vi "Timeout.vi"(8 "error in (no error)":errorcluster, 11 "State Machine Actor in":refnum<class "State Machine Actor.lvclass">) -> (0 "error out":errorcluster, 3 "State Machine Actor out":refnum<class "State Machine Actor.lvclass">)   [LabVIEW 2024, in "State Machine Actor.lvlib" / "State Machine Actor.lvclass"]
uses:
  State Machine Actor.lvclass
  State Machine Actor.lvclass/State Machine Actor.ctl
  <vilib>/ActorFramework/Actor/Actor.lvclass/Actor.ctl
  <vilib>/ActorFramework/Message Enqueuer/Message Enqueuer.lvclass/Message Enqueuer.ctl
  _State Machine Actor/_State Machine Actor/_State Machine Actor.lvclass
  Timed Out/Timed Out/Timed Out.lvclass
  <vilib>/ActorFramework/Actor/Actor.lvclass
  <vilib>/ActorFramework/Message Enqueuer/Message Priority.ctl
  <vilib>/ActorFramework/Message Enqueuer/Message Enqueuer.lvclass
  State Machine Actor Messages/Timeout Msg/Timeout Msg.lvclass
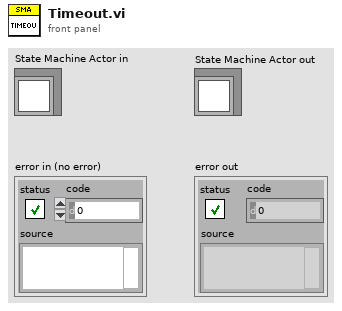
[diagram p1: front panel]
types:
  T1 = typedef "Actor Framework.lvlib/Message Enqueuer.lvclass/Message Priority.ctl" = enum16{"Low", "Normal", "High"}
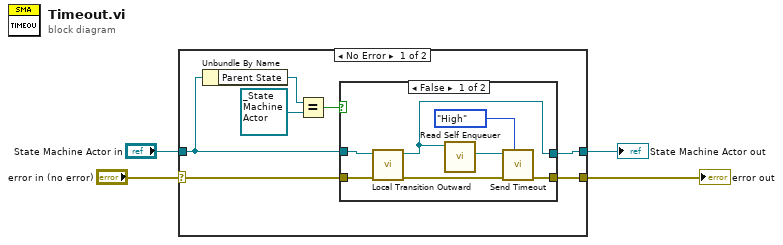
[diagram p0: block diagram]
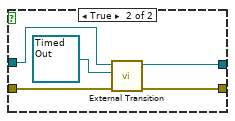
[diagram p2: hidden frame]
diagram:
  n1 = case shown="No Error" "error in (no error)" {
    selector: "error in (no error)" -> [w5 w25]
    tunnel: "State Machine Actor in" -> [w8 w24]
    tunnel: [w7 w24] -> w1
    tunnel: [w6 w25] -> w3
    frame No Error {
      n2 = Unbundle By Name(w8) -> ("Parent State"=w11:refnum<class "_State Machine Actor.lvclass">)
      n3 = Equal?(x=w11, y=refnum<class "_State Machine Actor.lvclass"> refnum ("Parent State")) -> (x = y?=w9:bool)
      n4 = case shown="False" w9 {
        tunnel: w8 -> [w18 w23]
        tunnel: [w17 w21] -> w7
        tunnel: w5 -> [w16 w20]
        tunnel: [w12 w19] -> w6
        frame False {
          n5 = call-dynamic "Local Transition Outward.vi"("error in (no error)"=w16, "State Machine Actor in"=w18) -> ("error out"=w13:errorcluster, "State Machine Actor out"=w17:refnum<class "State Machine Actor.lvclass">)  [unwired: 8 in]
          n6 = call <vilib>:"Read Self Enqueuer.vi"("Actor"=w17) -> ("Self Enqueuer"=w15:refnum<class "Message Enqueuer.lvclass">)  [unwired: 10 in]
          n7 = call "Send Timeout.vi"("Message Priority (Normal)"=Message_Priority."High", "error in (no error)"=w13, "Message Enqueuer"=w15) -> ("error out"=w12:errorcluster)  [unwired: 7 in, 1 out]
        }
        frame True {
          n8 = call-dynamic "External Transition.vi"("error in (no error)"=w20, "Target State in"=refnum<class "Timed Out.lvclass"> refnum ("Timed Out.lvlib:Timed Out.lvclass"), "State Machine Actor in"=w23) -> ("error out"=w19:errorcluster, "State Machine Actor out"=w21:refnum<class "State Machine Actor.lvclass">)  [unwired: 7 in]
        }
      }
    }
    frame Error {
    }
  }
  "error out" <- w3
  "State Machine Actor out" <- w1
